vi "Nested Case Structures Signum Function.vi"() -> ()   [LabVIEW 2019]
panel:
  out "Chart":i32(graph)
  in  "Push button to stop program":bool
  in  "Use slide to input number":dbl(slide) scale=-10.0..10.0
  # "Challenge: \nWrite a signum function that displays the results on a chart, returning +1 if the number is positive, -1 if the answer is negative, and 0 if the number is 0."
  # "Try it: Run the program and use the slide to input numbers."
  # "You will probably need:\nNested case structures, waveform chart, comparisons"
  # "Open the block diagram to see a possible solution."
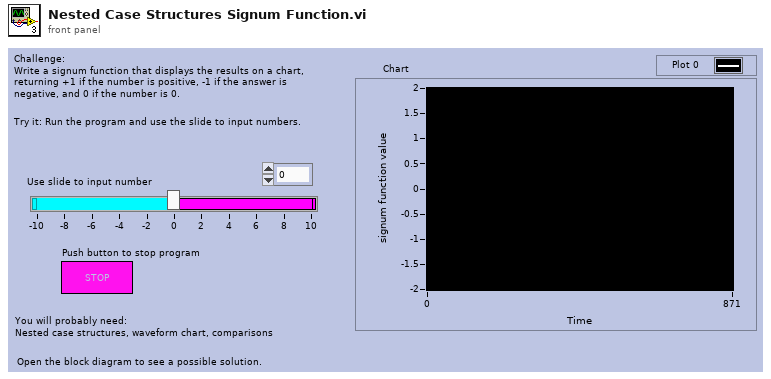
[diagram p1: front panel]
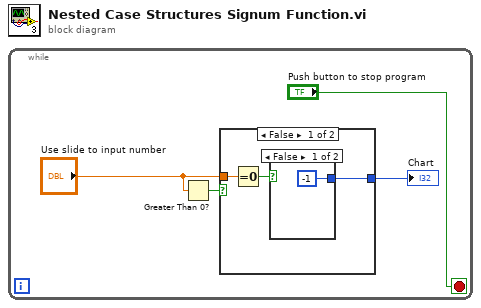
[diagram p0: block diagram]
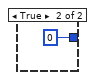
[diagram p2: hidden frame]
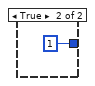
[diagram p3: hidden frame]
diagram:
  n1 = while {
    stop <- "Push button to stop program" stop-if-true
    n2 = Greater Than 0?(x="Use slide to input number") -> (x > 0?=w3:bool)
    n3 = case shown="False" w3 {
      tunnel: "Use slide to input number" -> [w7 _]
      tunnel: [w5 1] -> w1
      frame False {
        n4 = Equal To 0?(x=w7) -> (x = 0?=w6:bool)
        n5 = case shown="False" w6 {
          tunnel: [-1 0] -> w5
          frame False {
          }
          frame True {
          }
        }
      }
      frame True {
      }
    }
    "Chart" <- w1
  }
